vi "Log_Msg_Sub_VI.vi"(8 "error in (no error)":errorcluster, 10 "String":string, 11 "Byte Stream File in":refnum<file>) -> (0 "error out":errorcluster, 3 "Byte Stream File out":refnum<file>)   [LabVIEW 2017]
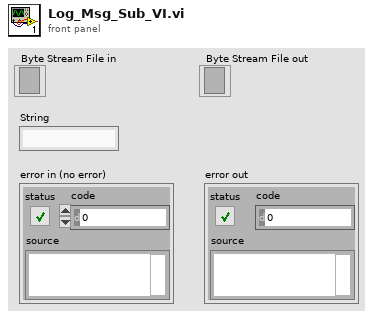
[diagram p1: front panel]
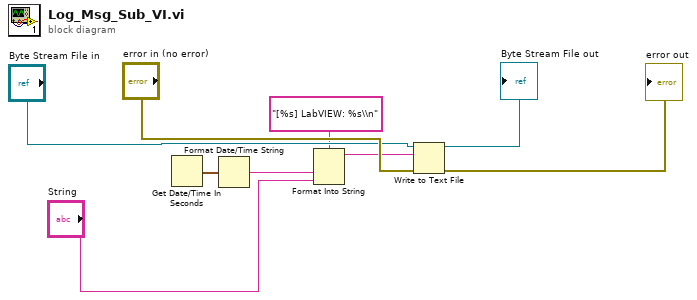
[diagram p0: block diagram]
diagram:
  n1 = Get Date/Time In Seconds() -> (seconds since 1Jan1904=w2:timestamp)
  n2 = Format Date/Time String(seconds (now)=w2) -> (date/time string=w4:string)  [unwired: 2 out]
  n3 = Format Into String(format string="[%s] LabVIEW: %s\\n", w4, "String") -> (resulting string=w5:string)  [unwired: 2 in, 1 out]
  n4 = Write to Text File(file (use dialog)="Byte Stream File in", text=w5, error in="error in (no error)") -> (refnum out=→"Byte Stream File out":refnum<file>, error out=→"error out":errorcluster)  [unwired: 2 out]
